vi "TrueCounterWReset.vi"(6 "Reset":bool, 9 "True?":bool) -> (1 "True Count":u16)   [LabVIEW 2010, in "kevLib2011.lvlib"]
doc: "Counts number of trues everytime it is run"
uses:
  kevLib2011.lvlib
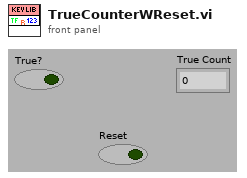
[diagram p1: front panel]
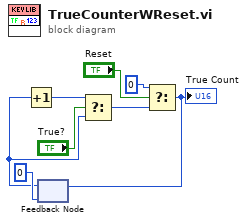
[diagram p0: block diagram]
diagram:
  n1 = feedback #1(u16 0 ("Mismatch Tol")) -> (w7:u16)
  n2 = Increment(x=w7) -> (x+1=w6:u16)
  n3 = Select(t=w6, s="True?", f=w7) -> (s? t:f=w3:u16)
  n4 = Select(t=u16 0, s="Reset", f=w3) -> (s? t:f=w1:u16)
  "True Count" <- w1
  n5 = feedback-in #1(w1) -> ()
